vi "motorFunctionWithReadout.vi"(0 "VISA Refnum in":refnum<visa-resource-name>, 1 "Fans":i32, 2 "zone 3 co2":dbl, 3 "zone 2 return":dbl, 4 "Light 1":i32, 5 "zone 2 co2":dbl, 6 "Light 3":i32, 7 "error in (no error)":errorcluster, 8 "zone 2 inlet":dbl, 9 "zone 3 inlet":dbl, 10 "zone 1 co2":dbl, 11 "Light 2":i32, 12 "zone 1 return":dbl, 13 "zone 3 return":dbl, 14 "zone 1 inlet":dbl, 16 "fresh air":dbl) -> (18 "String":string, 20 "VISA Refnum out":refnum<visa-resource-name>, 27 "error out":errorcluster)   [LabVIEW 2019]
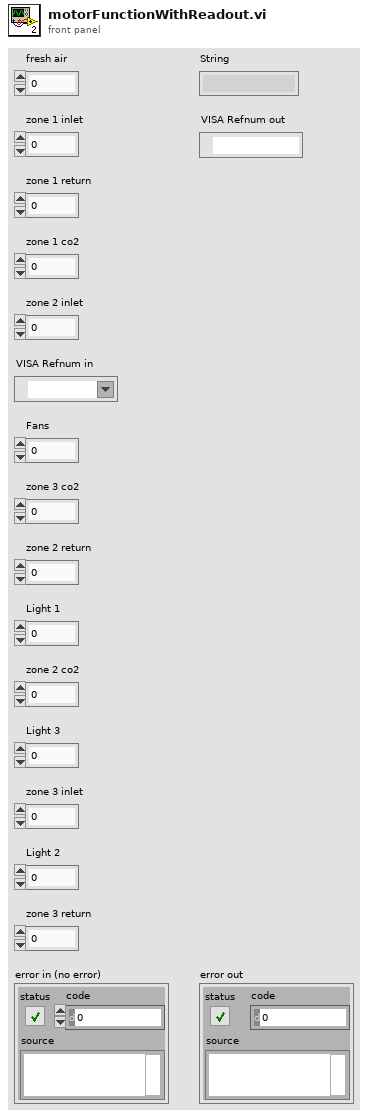
[diagram p1: front panel]
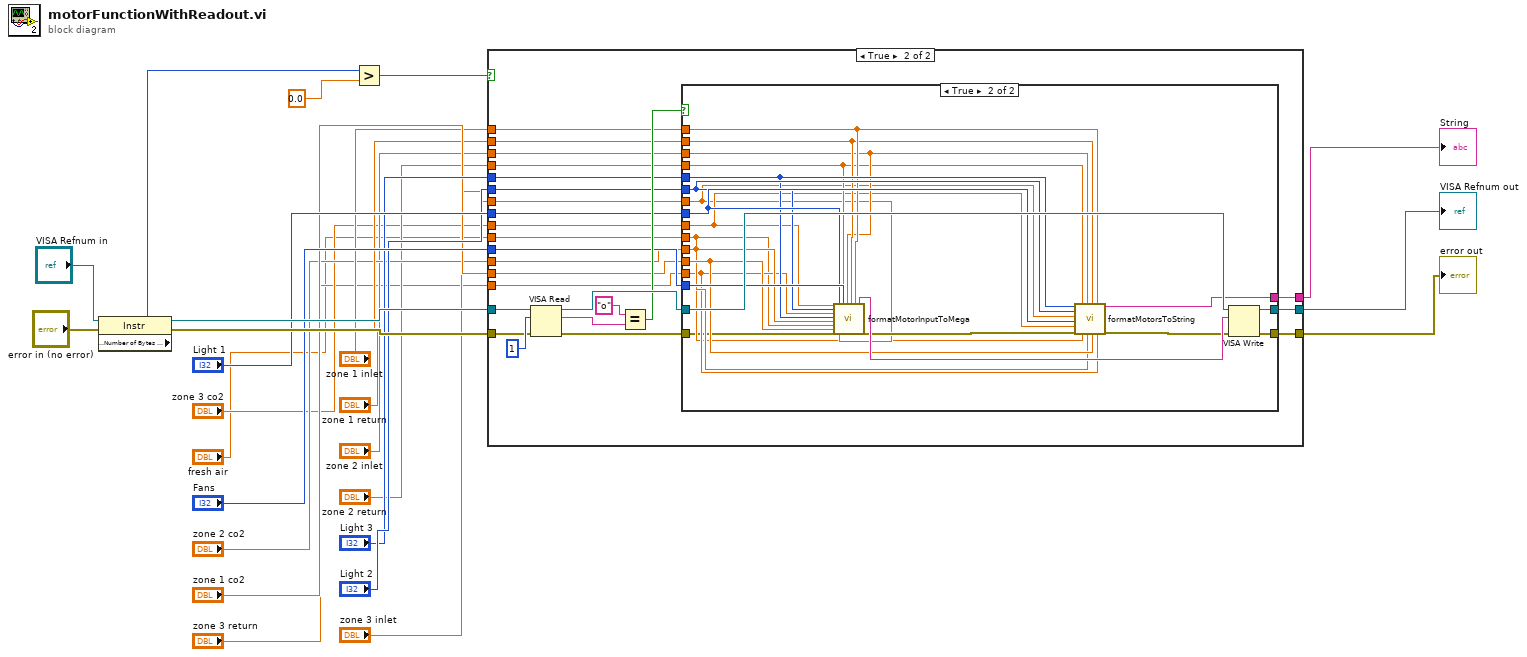
[diagram p0: block diagram]
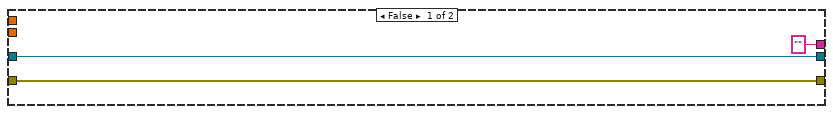
[diagram p2: hidden frame]
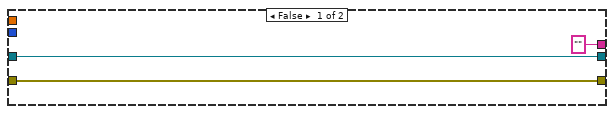
[diagram p3: hidden frame]
diagram:
  n1 = property class="Instr"(reference="VISA Refnum in", error in="error in (no error)") -> (reference out=w21:refnum<visa-resource-name>, error out=w20:errorcluster, "Serial Settings:Number of Bytes at Serial Port"=w23:u32)
  n2 = Greater?(x=w23, y=0.0) -> (0:w22:bool)
  n3 = case shown="True" w22 {
    tunnel: [w26 w51] -> w18
    tunnel: [w27 w50] -> w19
    tunnel: w21 -> [w26 w44]
    tunnel: w20 -> [w27 w43]
    tunnel: ["" ("String") w42] -> w15
    tunnel: "Fans" -> [_ w41]
    tunnel: "Light 1" -> [_ w40]
    tunnel: "Light 2" -> [_ w39]
    tunnel: "Light 3" -> [_ w38]
    tunnel: "zone 1 co2" -> [_ w37]
    tunnel: "zone 1 inlet" -> [_ w36]
    tunnel: "zone 1 return" -> [_ w35]
    tunnel: "zone 2 co2" -> [_ w34]
    tunnel: "zone 2 inlet" -> [_ w33]
    tunnel: "zone 2 return" -> [_ w32]
    tunnel: "zone 3 co2" -> [_ w31]
    tunnel: "zone 3 inlet" -> [_ w30]
    tunnel: "zone 3 return" -> [_ w29]
    tunnel: "fresh air" -> [_ w28]
    frame False {
    }
    frame True {
      n4 = VISA Read(VISA resource name=w44, byte count=u32 1, error in (no error)=w43) -> (VISA resource name out=w52:refnum<visa-resource-name>, read buffer=w46:string, error out=w49:errorcluster)  [unwired: 1 out]
      n5 = Equal?(x="o" ("y"), y=w46) -> (x = y?=w48:bool)
      n6 = case shown="True" w48 {
        tunnel: [w54 w77] -> w51
        tunnel: [w55 w76] -> w50
        tunnel: w49 -> [w55 w56]
        tunnel: w52 -> [w54 w75]
        tunnel: ["" ("String") w73] -> w42
        tunnel: w41 -> [_ w70]
        tunnel: w40 -> [_ w69]
        tunnel: w39 -> [_ w68]
        tunnel: w38 -> [_ w67]
        tunnel: w37 -> [_ w66]
        tunnel: w36 -> [_ w65]
        tunnel: w35 -> [_ w64]
        tunnel: w34 -> [_ w63]
        tunnel: w33 -> [_ w62]
        tunnel: w32 -> [_ w61]
        tunnel: w31 -> [_ w60]
        tunnel: w30 -> [_ w59]
        tunnel: w29 -> [_ w58]
        tunnel: w28 -> [_ w57]
        frame False {
        }
        frame True {
          n7 = call "formatMotorInputToMega.vi"("zone 3 co2"=w60, "Light in"=w68, "zone 3 return"=w58, "Light 3"=w67, "zone 2 co2"=w63, "fresh air"=w57, "zone 1 co2"=w66, "error in (no error)"=w56, "Light 1"=w69, "zone 3 inlet"=w59, "zone 2 return"=w61, "Fans"=w70, "zone 2 inlet"=w62, "zone 1 return"=w64, "zone 1 inlet"=w65) -> ("String"=w74:string, "error out"=w71:errorcluster)  [unwired: 11 in]
          n8 = call "formatMotorsToString.vi"("Light 3"=w67, "Light 2"=w68, "zone 3 inlet"=w59, "Light 1"=w69, "zone 3 co2"=w60, "error in (no error)"=w71, "zone 2 return"=w61, "fresh air"=w57, "zone 2 inlet"=w62, "zone 2 co2"=w63, "zone 1 return"=w64, "zone 1 co2"=w66, "zone 1 inlet"=w65, "zone 3 return"=w58) -> ("String"=w73:string, "error out"=w72:errorcluster)  [unwired: 4 in]
          n9 = VISA Write(VISA resource name=w75, write buffer=w74, error in (no error)=w72) -> (VISA resource name out=w77:refnum<visa-resource-name>, error out=w76:errorcluster)  [unwired: 1 out]
        }
      }
    }
  }
  "String" <- w15
  "error out" <- w19
  "VISA Refnum out" <- w18
